vi "LIA Test Frequency Shift Host.vi"() -> ()   [LabVIEW 2017]
uses:
  <vilib>/userdefined/Silver/nirio_resource_slv.ctl
  <vilib>/Analysis/4window.llb/windowTd.ctl
  <vilib>/Analysis/2dsp.llb/Complex FFT.vi
  <vilib>/FPGAPlugInAG/PXIe-7976R/niLvFpga_Open_PXIe-7976R.vi
  <vilib>/rvi/interface/common/dynamic/niFpgaDynamicAddResources.vi
  <vilib>/Utility/error.llb/Error Cluster From Error Code.vi
  <vilib>/rvi/errors/niLvFpgaAdjustHostInterfaceError.vi
  <vilib>/rvi/interface/common/niFpgaWaitOnOcc.vi
  <instrlib>/_niInstr/Streaming/v1/Host/Public/Start Continuous Stream.vi
  <vilib>/Analysis/0measdsp.llb/Scaled Time Domain Window (CDB).vi
  <vilib>/FPGAPlugInAG/Dynamic/niLvFpga_Close_Dynamic.vi
  <vilib>/rvi/interface/nirviOpenFPGA/nirviOpenFPGA.xnode
  FPGA Bitfiles/LIA Test Frequency Shift.lvbitx
  <vilib>/rvi/interface/nirviReadWriteControl/nirviReadWriteControl.xnode
  <vilib>/rvi/interface/nirviMethod/nirviMethod.xnode
  <vilib>/ErrorRing/Error Ring.xnode
  <vilib>/rvi/interface/nirviCloseFPGA/nirviCloseFPGA.xnode
  <instrlib>/_niInstr/Streaming/v1/Host/niInstr Streaming v1 Host.lvlib
  <vilib>/rvi/errors/niLvFpgaMergeErrorWithErrorCode.vi
  <vilib>/rvi/interface/Simulation/niFpgaSimulationCallBeginRW.vi
  <vilib>/FPGAPlugInAG/Dynamic/niLvFpga_ReadFifo_Dynamic.vi
  <vilib>/measure/NI_MAPro.lvlib
  <vilib>/FPGAPlugInAG/Dynamic/niLvFpga_StopFifo_Dynamic.vi
  <vilib>/FPGAPlugInAG/Dynamic/niLvFpga_ConfigureFifo_Dynamic.vi
  <vilib>/FPGAPlugInAG/Dynamic/niLvFpga_StartFifo_Dynamic.vi
  NiFpgaLv.dll
  <vilib>/Analysis/NI_AALPro.lvlib
  <vilib>/measure/maspectr.llb/FFT Power Spectrum and PSD for 1 Chan (CDB).vi
panel:
  out "Records Processed":i32
  out "Records Read":i32
  in  "Frequency Shift(Hz)":dbl=1000000.0 format="%#_p"
  out "Actual Depth":u32 format="%.0p"
  out "Samples Transferred":u64
  out "Power Specturm Graph":dbl[](graph)
  out "frequency shift":fxp<+/-,48,0> format="%.48g"
  out "nco frequency 0":fxp<+/-,48,0> format="%.48g"
  in  "Frequency (Hz)":dbl=1000000.0 format="%#_p"
  in  "Sampling Rate (Hz)":dbl=120000000.0 format="%#_p"
  out "Waveform Graph IQ":dbl[][](graph)
  in  "Number of Elements":u32=1200
  in  "Stop Button":bool
  out "error out":errorcluster
  in  "error in":errorcluster
  in  "Resource Name":T1="PXI2Slot2"
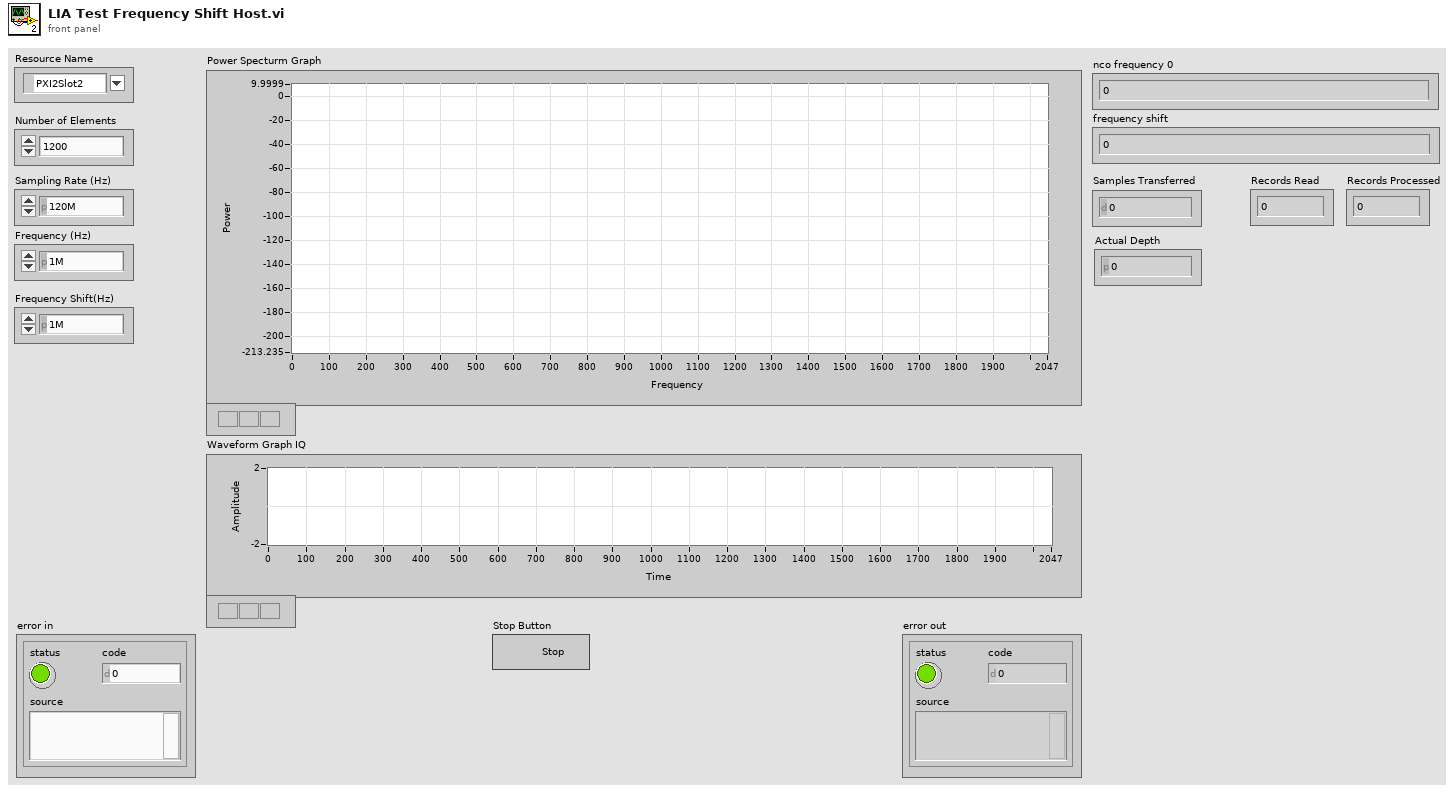
[diagram p1: front panel]
types:
  T1 = typedef "nirio_resource_slv.ctl" = tag
  T2 = typedef "niInstr Streaming v1 Common.lvlib/Stream State.ctl" = enum8{"Idle", "Finite Transfer", "Continuous", "Done", "Error", "Not Ready", "Cancel"}
  T3 = typedef "NI_AALPro.lvlib/windowTd.ctl" = u32
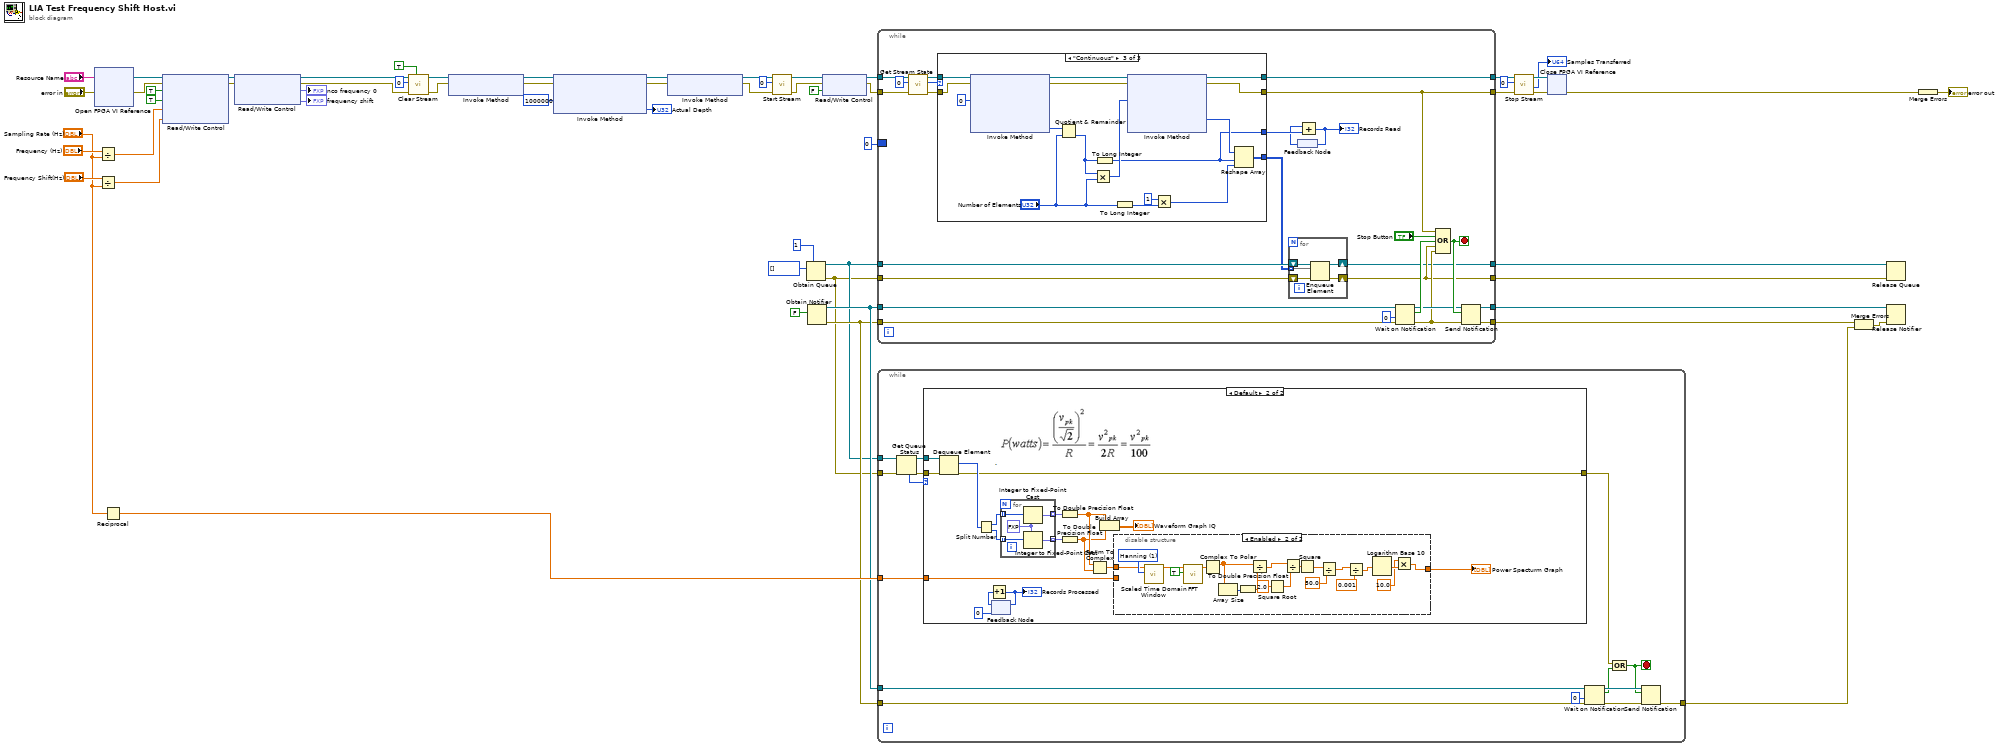
[diagram p0: block diagram]
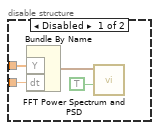
[diagram p3: hidden frame]
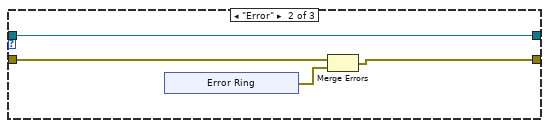
[diagram p5: hidden frame]
diagram:
  n1 = xnode "Open FPGA VI Reference"("error in"="error in", "resource name"="Resource Name") -> ("FPGA VI Reference Out"=w41:refnum<k20>, "error out"=w56:errorcluster)
  n2 = Divide(x="Frequency (Hz)", y="Sampling Rate (Hz)") -> (x/y=w37:dbl)
  n3 = Divide(x="Frequency Shift(Hz)", y="Sampling Rate (Hz)") -> (x/y=w18:dbl)
  n4 = Reciprocal(x="Sampling Rate (Hz)") -> (1/x=w16:dbl)
  n5 = xnode "Read/Write Control"("FPGA VI Reference In"=w41, "error in"=w56, "nco enable (T) 0"=TRUE ("reset"), "nco enable (T) 0"=TRUE ("nco enable (T)"), "nco frequency 0"=w37, "frequency shift 0"=w18) -> ("FPGA VI Reference Out"=w36:refnum<k20>, "error out"=w35:errorcluster)
  n6 = xnode "Read/Write Control"("FPGA VI Reference In"=w36, "error in"=w35) -> ("FPGA VI Reference Out"=w34:refnum<k20>, "error out"=w33:errorcluster, "nco frequency 0"=→"nco frequency 0":fxp<+/-,48,0>, "frequency shift 0"=→"frequency shift":fxp<+/-,48,0>)
  n7 = call <instrlib>:"Clear Stream.vi"("clear on error in?"=TRUE, "error in (no error)"=w33, "stream index"=0, "refnum in"=w34) -> ("error out"=w55:errorcluster, "refnum out"=w51:refnum<k20>)  [unwired: 6 in]
  n8 = xnode "Invoke Method"("FPGA VI Reference In"=w51, "error in"=w55) -> ("FPGA VI Reference Out"=w29:refnum<k20>, "error out"=w52:errorcluster)
  n9 = xnode "Invoke Method"("FPGA VI Reference In"=w29, "error in"=w52, "Requested Depth"=u32 1000000) -> ("FPGA VI Reference Out"=w28:refnum<k20>, "error out"=w30:errorcluster, "Actual Depth"=→"Actual Depth":u32)
  n10 = xnode "Invoke Method"("FPGA VI Reference In"=w28, "error in"=w30) -> ("FPGA VI Reference Out"=w49:refnum<k20>, "error out"=w50:errorcluster)
  n11 = call-poly <instrlib>:"Start Stream.vi"("error in (no error)"=w50, "stream index"=0, "refnum in"=w49) -> ("error out"=w47:errorcluster, "refnum out"=w44:refnum<k20>)  [unwired: 7 in]
  n12 = Obtain Queue(max queue size (-1, unlimited)=1, element data type=u64[] [] ("Data")) -> (queue out=w4:refnum<queue>, error out=w3:errorcluster)  [unwired: 3 in, 1 out]
  n13 = Obtain Notifier(notification data type=FALSE) -> (notifier out=w10:refnum<notifier>, error out=w9:errorcluster)  [unwired: 3 in, 1 out]
  n14 = xnode "Read/Write Control"("FPGA VI Reference In"=w44, "error in"=w47, "reset (T) 0"=FALSE ("reset")) -> ("FPGA VI Reference Out"=w43:refnum<k20>, "error out"=w45:errorcluster)
  n15 = while {
    tunnel: [w82] -> w25
    tunnel: w43 -> [w81]
    tunnel: [w84] -> w26
    tunnel: w45 -> [w79]
    tunnel: [w74] -> w14
    tunnel: w10 -> [w72]
    tunnel: [w75] -> w13
    tunnel: w9 -> [w71]
    tunnel: [w63] -> w6
    tunnel: w4 -> [w64]
    tunnel: [w65] -> w5
    tunnel: w3 -> [w67]
    border: 0 -> [_]
    stop <- w73 stop-if-true
    n16 = call <instrlib>:"Get Stream State.vi"("error in (no error)"=w79, "stream index"=0, "refnum in"=w81) -> ("error out"=w78:errorcluster, "stream state"=w77:T2, "refnum out"=w80:refnum<k20>)  [unwired: 6 in]
    n17 = case shown="\"Continuous\"" w77 {
      tunnel: [w90 w93 w107] -> w84
      tunnel: [w91 w95 w106] -> w82
      tunnel: w80 -> [w91 w95 w105]
      tunnel: w78 -> [w90 w94 w104]
      tunnel: [_ _ w103] -> w62
      tunnel: [_ _ w101] -> w61
      frame Default {
      }
      frame "Error" {
        n18 = xnode "Error Ring"() -> ("error out"=w92:errorcluster)
        n19 = Merge Errors(w94, w92) -> (w93:errorcluster)
      }
      frame "Continuous" {
        n20 = xnode "Invoke Method"("FPGA VI Reference In"=w105, "error in"=w104, "Number of Elements"=u32 0) -> ("FPGA VI Reference Out"=w113:refnum<k20>, "error out"=w114:errorcluster, "Elements Remaining"=w112:u32)  [unwired: 1 in, 1 out]
        n21 = Quotient & Remainder(x=w112, y="Number of Elements") -> (floor(x/y)=w102:u32)  [unwired: 1 out]
        n22 = Multiply(x=w102, y="Number of Elements") -> (x*y=w116:u32)
        n23 = To Long Integer(number=w102) -> (32bit integer=w101:i32)
        n24 = To Long Integer(number="Number of Elements") -> (32bit integer=w115:i32)
        n25 = xnode "Invoke Method"("FPGA VI Reference In"=w113, "error in"=w114, "Number of Elements"=w116) -> ("FPGA VI Reference Out"=w106:refnum<k20>, "error out"=w107:errorcluster, "Data"=w117:u64[])  [unwired: 1 in, 1 out]
        n26 = Multiply(x=1, y=w115) -> (x*y=w108:i32)
        n27 = Reshape Array(w117, w101, w108) -> (w103:u64[][])
      }
    }
    n28 = for {
      shift-right: [w88] -> w65
      shift-left: w67 -> [w89]
      shift-right: [w86] -> w63
      shift-left: w64 -> [w87]
      tunnel: w62 -> [w85] mode=indexing
      n29 = Enqueue Element(queue=w87, element=w85, error in (no error)=w89) -> (queue out=w86:refnum<queue>, error out=w88:errorcluster)  [unwired: 1 in, 1 out]
    }
    n30 = feedback #1() -> (w60:i32)
    n31 = Add(x=w60, y=w61) -> (x+y=w59:i32)
    "Records Read" <- w59
    n32 = feedback-in #1(w59) -> ()
    n33 = Wait on Notification(notifier=w72, timeout in ms (-1)=0, error in (no error)=w71) -> (notifier out=w68:refnum<notifier>, notification=w69:bool, error out=w66:errorcluster)  [unwired: 1 in, 1 out]
    n34 = Compound Arithmetic op=OR(w84, "Stop Button", w69, w65, w66) -> (w73:bool)
    n35 = Send Notification(notification=w73, notifier=w68, error in (no error)=w66) -> (notifier out=w74:refnum<notifier>, error out=w75:errorcluster)
  }
  n36 = while {
    tunnel: w16 -> [w132]
    tunnel: [w126] -> w11
    tunnel: w10 -> [w125]
    tunnel: w9 -> [w124]
    tunnel: w4 -> [w121]
    tunnel: w3 -> [w123]
    stop <- w127 stop-if-true
    n37 = Get Queue Status(queue=w121, error in (no error)=w123) -> (queue out=w120:refnum<queue>, error out=w122:errorcluster, # elements in queue=w119:i32)  [unwired: 1 in, 5 out]
    n38 = case shown="Default" w119 {
      tunnel: w132 -> [_ w150]
      tunnel: w122 -> [w133 w148]
      tunnel: w120 -> [_ w147]
      tunnel: [w133 w146] -> w118
      frame 0 {
      }
      frame Default {
        n39 = Dequeue Element(queue=w147, error in (no error)=w148) -> (element=w149:u64[], error out=w146:errorcluster)  [unwired: 1 in, 2 out]
        n40 = Split Number(x=w149) -> (hi(x)=w143:u32[], lo(x)=w142:u32[])
        n41 = feedback #2(0) -> (w144:i32)
        n42 = Increment(x=w144) -> (x+1=w145:i32)
        "Records Processed" <- w145
        n43 = feedback-in #2(w145) -> ()
        n44 = for {
          tunnel: w143 -> [w179] mode=indexing
          tunnel: w142 -> [w178] mode=indexing
          tunnel: [w176] -> w141 mode=indexing
          tunnel: [w175] -> w140 mode=indexing
          w177 = fxp<+/-,32,16> 0.0 ("fixed-point type")
          n45 = Integer to Fixed-Point Cast(fixed-point type=w177, integer=w179) -> (fixed-point=w176:fxp<+/-,32,16>)
          n46 = Integer to Fixed-Point Cast(fixed-point type=w177, integer=w178) -> (fixed-point=w175:fxp<+/-,32,16>)
        }
        n47 = To Double Precision Float(number=w141) -> (double precision float=w138:dbl[])
        n48 = To Double Precision Float(number=w140) -> (double precision float=w137:dbl[])
        n49 = Re/Im To Complex(1:w137, 2:w138) -> (0:w134:cdb[])
        n50 = Build Array(w138, w137) -> (→"Waveform Graph IQ":dbl[][])
        n51 = disable-structure shown="Enabled" {
          disable-tunnel: w150 -> [w154 _]
          disable-tunnel: w134 -> [w153 w156]
          disable-tunnel: [_ w167] -> w135
          frame Disabled {
            n52 = Bundle By Name("Y"=w153, "dt"=w154) -> (w152:waveform(cdb))  [unwired: 1 in]
            n53 = call-poly <vilib>:"FFT Power Spectrum and PSD.vi"("dB On (F)"=TRUE, "time signal"=w152) -> ()  [unwired: 6 in, 4 out]
          }
          frame Enabled {
            w157 = T3 1 items=["Rectangle"=0, "Hanning"=1, "Hamming"=2, "Blackman-Harris"=3, "Exact Blackman"=4, "Blackman"=5, "Flat Top"=6, "4 Term B-Harris "=7, "7 Term B-Harris"=8, "Low Sidelobe"=9, "Blackman Nuttall"=11, "Triangle"=30, "Bartlett-Hanning"=31, "Bohman"=32, "Parzen"=33, "Welch"=34, "Kaiser"=60, "Dolph-Chebyshev"=61, "Gaussian"=62] ("window")
            n54 = call-poly <vilib>:"Scaled Time Domain Window.vi"("window"=w157, "X"=w156) -> ("Windowed X"=w155:cdb[])  [unwired: 7 in, 2 out]
            n55 = call-poly <vilib>:"FFT.vi"("shift?"=TRUE, "X"=w155) -> ("FFT {X}"=w174:cdb[])  [unwired: 8 in, 1 out]
            n56 = Complex To Polar(r * e^(i*theta)=w174) -> (r=w172:dbl[])  [unwired: 1 out]
            n57 = Array Size(array=w172) -> (size(s)=w171:i32)
            n58 = To Double Precision Float(number=w171) -> (double precision float=w162:dbl)
            n59 = Divide(x=w172, y=w162) -> (x/y=w173:dbl[])
            n60 = Square Root(x=2.0) -> (sqrt(x)=w160:dbl)
            n61 = Divide(x=w173, y=w160) -> (x/y=w158:dbl[])
            n62 = Square(x=w158) -> (x^2=w170:dbl[])
            n63 = Divide(x=w170, y=50.0) -> (x/y=w165:dbl[])
            n64 = Divide(x=w165, y=0.001) -> (x/y=w159:dbl[])
            n65 = Logarithm Base 10(1:w159) -> (0:w168:dbl[])
            n66 = Multiply(x=10.0, y=w168) -> (x*y=w167:dbl[])
          }
        }
        "Power Specturm Graph" <- w135
      }
    }
    n67 = Wait on Notification(notifier=w125, timeout in ms (-1)=0, error in (no error)=w124) -> (notifier out=w130:refnum<notifier>, notification=w128:bool, error out=w131:errorcluster)  [unwired: 1 in, 1 out]
    n68 = Compound Arithmetic op=OR(w118, w128) -> (w127:bool)
    n69 = Send Notification(notification=w127, notifier=w130, error in (no error)=w131) -> (error out=w126:errorcluster)  [unwired: 1 out]
  }
  n70 = call <instrlib>:"Stop Stream.vi"("error in (no error)"=w26, "stream index"=0, "refnum in"=w25) -> ("error out"=w23:errorcluster, "samples transferred"=→"Samples Transferred":u64, "refnum out"=w24:refnum<k20>)  [unwired: 5 in, 1 out]
  n71 = xnode "Close FPGA VI Reference"("FPGA VI Reference In"=w24, "error in"=w23) -> ("error out"=w46:errorcluster)
  n72 = Merge Errors(w13, w11) -> (w12:errorcluster)
  n73 = Release Queue(queue=w6, error in (no error)=w5) -> ()  [unwired: 1 in, 3 out]
  n74 = Release Notifier(notifier=w14, error in (no error)=w12) -> ()  [unwired: 1 in, 3 out]
  n75 = Merge Errors(w46) -> (→"error out":errorcluster)
